vi "Directory of Top Level VI (excel).vi"(0 "error in (no error)":errorcluster) -> (1 "directory of top VI":path, 2 "error out":errorcluster)   [LabVIEW 2010, in "NI_ReportGenerationToolkit.lvlib"]
doc: "This VI will get the directory in which the top level VI of the program is contained. If VI is in a library (.llb) file the directory in which the library file exists is returned"
uses:
  <vilib>/addons/_office/NI_ReportGenerationToolkit.lvlib
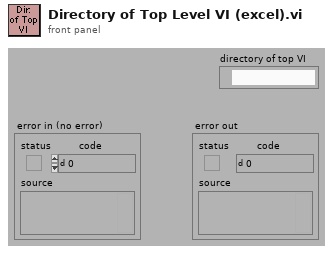
[diagram p1: front panel]
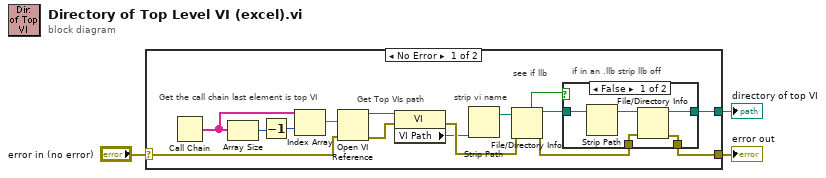
[diagram p0: block diagram]
diagram:
  n1 = case shown="No Error" "error in (no error)" {
    selector: "error in (no error)" -> [w4 w26]
    tunnel: [w18 _] -> w3
    tunnel: [w5 w26] -> w2
    frame No Error {
      # "see if llb"
      # "strip vi name"
      # "Get Top VIs path"
      # "Get the call chain last element is top VI"
      # "if in an .llb strip llb off"
      n2 = Call Chain() -> (call chain=w9:string[])
      n3 = Array Size(array=w9) -> (size(s)=w7:i32)
      n4 = Decrement(x=w7) -> (x-1=w8:i32)
      n5 = Index Array(array=w9, index=w8) -> (element=w10:string)
      n6 = Open VI Reference(vi path=w10, error in (no error)=w4) -> (vi reference=w11:refnum<vi>, error out=w15:errorcluster)  [unwired: 4 out]
      n7 = property class="VI"(reference=w11, error in=w15) -> (error out=w17:errorcluster, "VI Path"=w16:path)  [unwired: 1 out]
      n8 = Strip Path(path=w16) -> (stripped path=w12:path)  [unwired: 1 out]
      n9 = File/Directory Info(path=w12, error in=w17) -> (path out=w14:path, directory=w13:bool, error out=w6:errorcluster)  [unwired: 4 out]
      n10 = case shown="False" w13 {
        tunnel: w14 -> [w23 w25]
        tunnel: [w19 w25] -> w18
        tunnel: w6 -> [w21 w24]
        tunnel: [w20 w24] -> w5
        frame False {
          n11 = Strip Path(path=w23) -> (stripped path=w22:path)  [unwired: 1 out]
          n12 = File/Directory Info(path=w22, error in=w21) -> (path out=w19:path, error out=w20:errorcluster)  [unwired: 5 out]
        }
        frame True {
        }
      }
    }
    frame Error {
    }
  }
  "error out" <- w2
  "directory of top VI" <- w3
